vi "GetTagName.vi"() -> (0 "OK":bool, 1 "Type":string, 2 "Name":string)   [LabVIEW 2016]
doc: "Displays a standard dialog box that prompts users to enter information, such as a user name and password.\n--------------------\n\nThis Express VI is configured as follows:\n\nMessage to Display to the User:Please enter the tag name and type (INT, DOUBLE or STRING)\nThe inputs are: \nText Entry Box: Name\nText Entry Box: Type"
panel:
  in  "type":string(combo)="STRING"
  in  "Name In":string caption="Name"
  in  "Create":bool caption="OK2"
  # "Please enter the tag name and type"
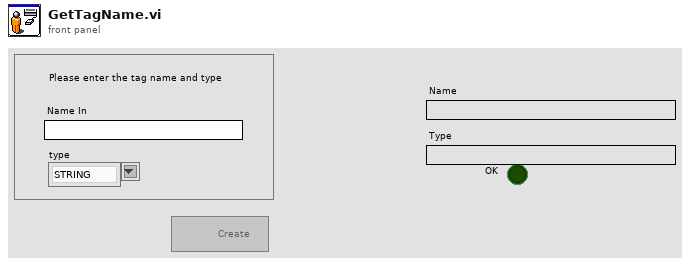
[diagram p1: front panel]
types:
  T1 = enum8{"Enabled", "Disabled", "Disabled and Grayed Out"}
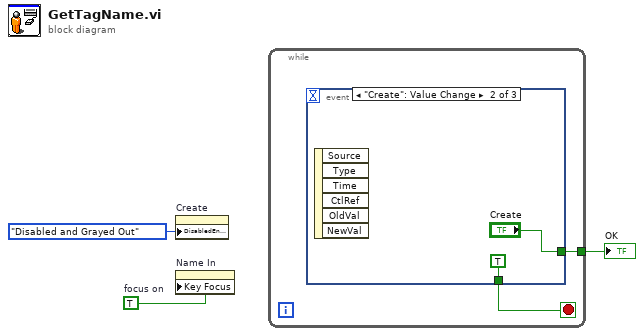
[diagram p0: block diagram]
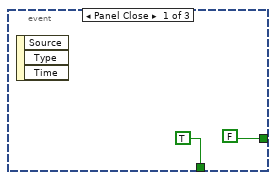
[diagram p2: hidden frame]
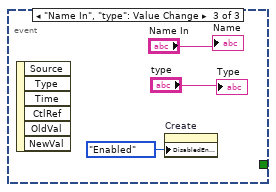
[diagram p3: hidden frame]
diagram:
  w3 = TRUE  # focus on
  n1 = property on="Create" class="Bool"("DisabledEnum"=T1."Disabled and Grayed Out" ("Disabled")) -> ()  [unwired: 2 in, 2 out]
  n2 = property on="Name In" class="Str"("Key Focus"=w3) -> ()  [unwired: 2 in, 2 out]
  n3 = while {
    tunnel: [w5] -> w2
    stop <- w4 stop-if-true
    n4 = event shown="[1] \"Create\": Value Change" {
      selector: _ -> [_ _ _]
      dyn-events: _ -> [_ _ _]
      timeout: _ -> [_ _ _]
      tunnel: [FALSE "Create" _] -> w5
      tunnel: [TRUE TRUE _] -> w4
      event Panel Close {
        n5 = event-data() -> ()  [unwired: 1 in, 3 out]
      }
      event "Create": Value Change {
        n6 = event-data() -> ()  [unwired: 1 in, 6 out]
      }
      event "Name In", "type": Value Change {
        n7 = event-data() -> ()  [unwired: 1 in, 6 out]
        n8 = property on="Create" class="Bool"("DisabledEnum"=T1."Enabled" ("Disabled")) -> ()  [unwired: 2 in, 2 out]
        "Name" <- "Name In"
        "Type" <- "type"
      }
    }
  }
  "OK" <- w2
